vi "Robot Main.vi"() -> ()   [LabVIEW 2019]
doc: "This VI implements the framework and scheduler for your robotics program. It should not be necessary to modify the framework. You are expected to add your code to the VIs called from Robot Main - the ones located in the Team Code folder within the project."
uses:
  <vilib>/Rock Robotics/SystemInterfaces/i2clib/i2c_bus.ctl
panel:
  out "Matched Color Name":string
  out "Match Confidence":dbl
  out "Measured Color":cluster{"R":dbl, "G":dbl, "B":dbl}
  in  "Blue Calibration":cluster{"R":dbl, "G":dbl, "B":dbl}={"R"=0.143, "G"=0.427, "B"=0.429}
  in  "Green Calibration":cluster{"R":dbl, "G":dbl, "B":dbl}={"R"=0.197, "G"=0.561, "B"=0.24}
  in  "Red Calibration":cluster{"R":dbl, "G":dbl, "B":dbl}={"R"=0.561, "G"=0.323, "B"=0.114}
  in  "Yellow Calibration":cluster{"R":dbl, "G":dbl, "B":dbl}={"R"=0.361, "G"=0.524, "B"=0.113}
  out "error out":errorcluster
  out "Proximity":u16(graph)
  out "Color":u32(colorbox)
  in  "I2C Bus":T1
  in  "Finish":bool
  # "Target Calibration (Latched at the start)"
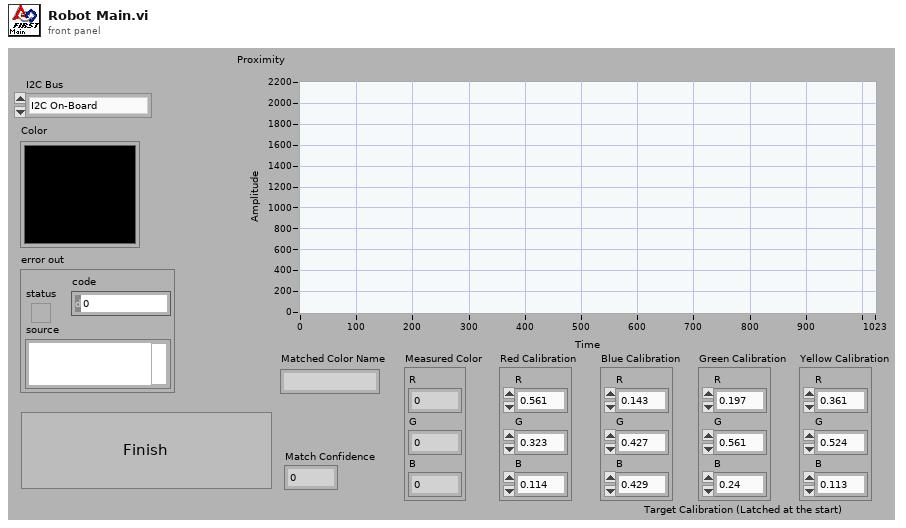
[diagram p1: front panel]
types:
  T1 = typedef "i2c_bus.ctl" = enum16{"I2C On-Board", "I2C MXP", "Invalid"}
  T2 = typedef "Color Sensor V3 DevRef.ctl" = cluster{"I2CDevRef":T3}
  T3 = typedef "WPI_I2CDevRef.ctl" = cluster{"DevStatus":errorcluster, "Device Address":u8, "Handle":i32, "I2C Bus":T1}
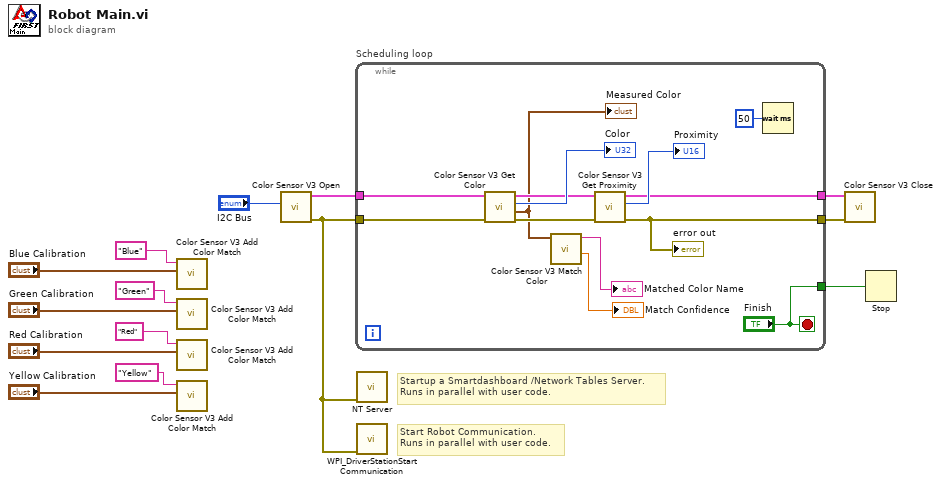
[diagram p0: block diagram]
diagram:
  # "Startup a Smartdashboard /Network Tables Server.\nRuns in parallel with user code."
  # "Start Robot Communication.\nRuns in parallel with user code."
  n1 = call <vilib>:"Color Sensor V3 Add Color Match.vi"("Color"="Blue Calibration", "Name"="Blue") -> ()  [unwired: 10 in]
  n2 = call <vilib>:"Color Sensor V3 Add Color Match.vi"("Color"="Green Calibration", "Name"="Green") -> ()  [unwired: 10 in]
  n3 = call <vilib>:"Color Sensor V3 Add Color Match.vi"("Color"="Red Calibration", "Name"="Red") -> ()  [unwired: 10 in]
  n4 = call <vilib>:"Color Sensor V3 Add Color Match.vi"("Color"="Yellow Calibration", "Name"="Yellow") -> ()  [unwired: 10 in]
  n5 = call <vilib>:"Color Sensor V3 Open.vi"("I2C Bus"="I2C Bus") -> ("error out"=w12:errorcluster, "ColorSensorDevRef"=w13:T2)  [unwired: 9 in]
  n6 = while "Scheduling loop" {
    tunnel: w13 -> [w21]
    tunnel: w12 -> [w20]
    tunnel: ["Finish"] -> w11
    tunnel: [w16] -> w2
    tunnel: [w15] -> w1
    stop <- "Finish" stop-if-true
    n7 = call <vilib>:"Color Sensor V3 Get Color.vi"("error in (no error)"=w20, "ColorSensorDevRef"=w21) -> ("error out"=w25:errorcluster, "Normalized Color"=w19:cluster{"R":dbl, "G":dbl, "B":dbl}, "Color"=→"Color":u32, "ColorSensorDevRef out"=w24:T2)  [unwired: 6 in]
    "Measured Color" <- w19
    n8 = call <vilib>:"Color Sensor V3 Match Color.vi"("Measured Color"=w19) -> ("Confidence"=→"Match Confidence":dbl, "Matched Color Name"=→"Matched Color Name":string)  [unwired: 8 in, 1 out]
    n9 = call <vilib>:"Color Sensor V3 Get Proximity.vi"("error in (no error)"=w25, "ColorSensorDevRef"=w24) -> ("error out"=w15:errorcluster, "Proximity"=→"Proximity":u16, "ColorSensorDevRef out"=w16:T2)  [unwired: 7 in]
    "error out" <- w15
    n10 = Wait (ms)(milliseconds to wait=u32 50) -> ()  [unwired: 1 out]
  }
  n11 = call <vilib>:"NT Server.vi"("error in (no error)"=w12) -> ()  [unwired: 11 in]
  n12 = call <vilib>:"WPI_DriverStationStart Communication.vi"("error in (no error)"=w12) -> ()  [unwired: 1 in, 10 out]
  n13 = call <vilib>:"Color Sensor V3 Close.vi"("error in (no error)"=w1, "ColorSensorDevRef in"=w2) -> ()  [unwired: 9 in, 1 out]
  n14 = Stop(stop? (T)=w11) -> ()
